vi "my ai2 and ai3 one shot on demand.vi"(0 "device name":tag="Dev1", 1 "timeout (s)":dbl=10.0 format="%0.2f", 2 "stop (T)":bool=TRUE, 11 "error in":errorcluster) -> (4 "task out":refnum<k21>, 6 "thermistor":dbl, 10 "heater":dbl, 15 "error out":errorcluster)   [LabVIEW 2019]
doc: "Creates, edits, and runs tasks using NI-DAQmx. Refer to the NI-DAQmx Readme for a complete listing of devices NI-DAQmx supports.\n\nWhen you place this Express VI on the block diagram, the DAQ Assistant launches to create a new task. After you create a task, you can double-click the DAQ Assistant Express VI to edit that task. For continuous measurement or generation, place a while loop around the DAQ Assistant Express VI."
uses:
  <vilib>/DAQmx/read.llb/DAQmx Read.vi
  <vilib>/DAQmx/read.llb/DAQmx Read (Analog 1D DBL NChan 1Samp).vi
  <vilib>/DAQmx/create/channels.llb/DAQmx Create Channel (TEDS-AI-Voltage-Basic).vi
  <vilib>/DAQmx/create/channels.llb/DAQmx Create Channel (AI-Voltage-Basic).vi
  <vilib>/DAQmx/miscellaneous.llb/DAQmx Fill In Error Info.vi
panel:
  out "data":dynamicdata(waveform)
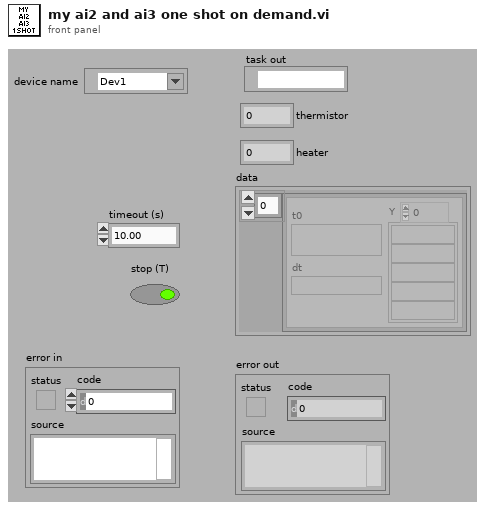
[diagram p1: front panel]
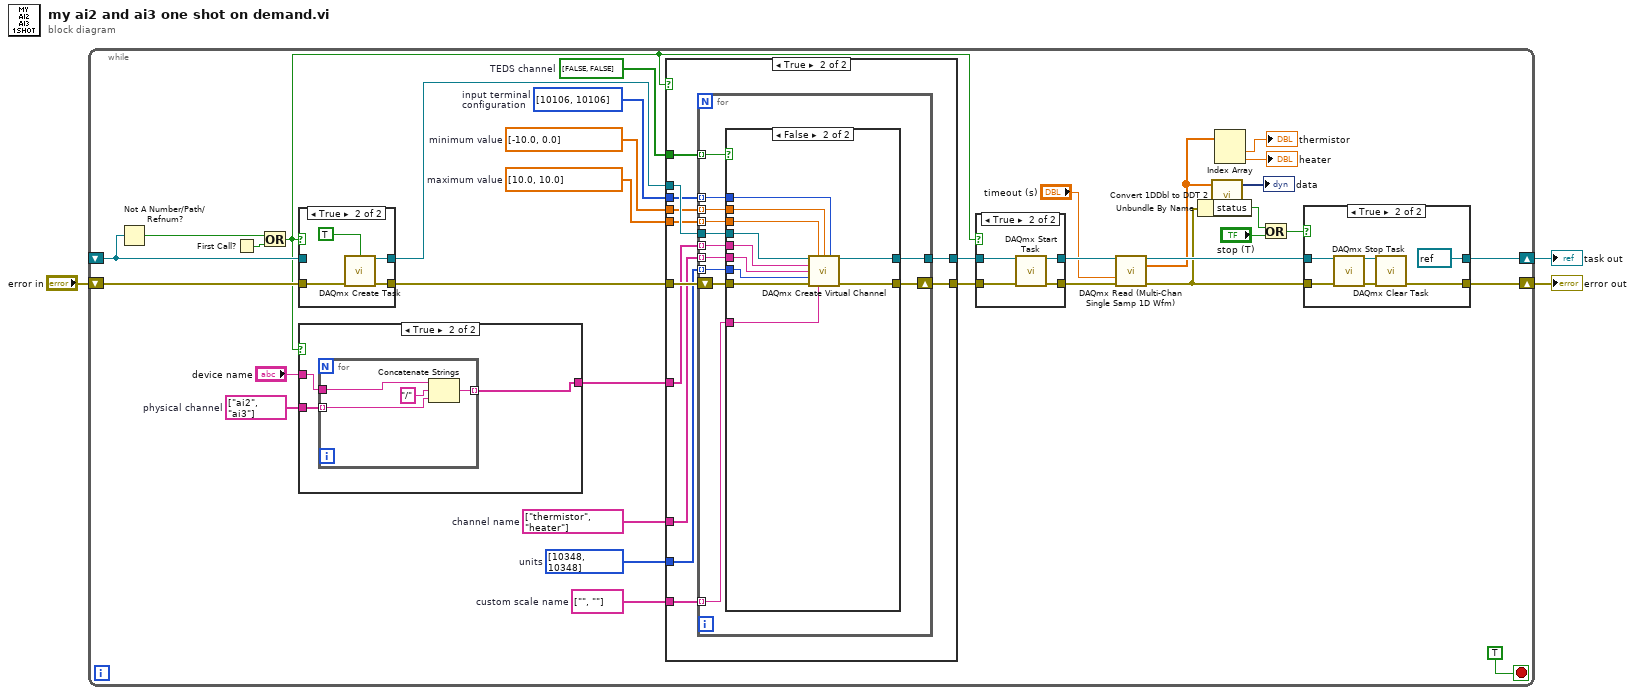
[diagram p0: block diagram]
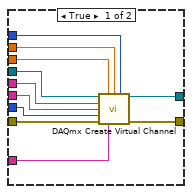
[diagram p5: hidden frame]
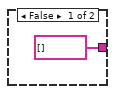
[diagram p6: hidden frame]
diagram:
  n1 = while {
    shift-right: [w13] -> w1
    shift-left: _ -> [w34]
    shift-right: [w11] -> w2
    shift-left: "error in" -> [w35]
    stop <- TRUE stop-if-true
    w21 = bool[] [FALSE, FALSE]  # TEDS channel
    w22 = string[] ["", ""]  # custom scale name
    w23 = i32[] [10348, 10348] items=["Volts"=10348, "From TEDS"=12516, "From Custom Scale"=10065]  # units
    w24 = string[] ["thermistor", "heater"]  # channel name
    w26 = dbl[] [10.0, 10.0]  # maximum value
    w27 = dbl[] [-10.0, 0.0]  # minimum value
    w28 = i32[] [10106, 10106] items=["default"=-1, "RSE"=10083, "NRSE"=10078, "Differential"=10106, "Pseudodifferential"=12529]  # input terminal configuration
    w31 = string[] ["ai2", "ai3"]  # physical channel
    n2 = Not A Number/Path/Refnum?(number/path/refnum=w34) -> (NaN/Path/Refnum?=w33:bool)
    n3 = First Call?() -> (First Call?: T/F=w36:bool)
    n4 = Or(x=w33, y=w36) -> (x .or. y?=w20:bool)
    n5 = case shown="True" w20 {
      tunnel: [w109 w113] -> w30
      tunnel: w34 -> [w109 _]
      tunnel: [w108 w112] -> w29
      tunnel: w35 -> [w108 w110]
      frame False {
      }
      frame True {
        n6 = call <vilib>:"DAQmx Create Task.vi"("auto cleanup"=TRUE, "error in"=w110) -> ("task out"=w113:refnum<k21>, "error out"=w112:errorcluster)  [unwired: 12 in]
      }
    }
    n7 = case shown="True" w20 {
      tunnel: [string[] [] w103] -> w25
      tunnel: "device name" -> [_ w102]
      tunnel: w31 -> [_ w101]
      frame False {
      }
      frame True {
        n8 = for {
          tunnel: [w107] -> w103 mode=indexing
          tunnel: w102 -> [w106]
          tunnel: w101 -> [w104] mode=indexing
          n9 = Concatenate Strings(w106, "/" ("string"), w104) -> (w107:string)
        }
      }
    }
    n10 = case shown="True" w20 {
      tunnel: [w53 w63] -> w19
      tunnel: w30 -> [w53 w65]
      tunnel: [w52 w62] -> w18
      tunnel: w29 -> [w52 w64]
      tunnel: w28 -> [_ w61]
      tunnel: w27 -> [_ w60]
      tunnel: w26 -> [_ w59]
      tunnel: w25 -> [_ w58]
      tunnel: w24 -> [_ w57]
      tunnel: w23 -> [_ w56]
      tunnel: w22 -> [_ w55]
      tunnel: w21 -> [_ w54]
      frame False {
      }
      frame True {
        n11 = for {
          tunnel: w65 -> [w77]
          tunnel: [w75] -> w63
          tunnel: w61 -> [w73] mode=indexing
          tunnel: w60 -> [w72] mode=indexing
          tunnel: w59 -> [w71] mode=indexing
          tunnel: w58 -> [w70] mode=indexing
          tunnel: w57 -> [w69] mode=indexing
          tunnel: w56 -> [w68] mode=indexing
          tunnel: w55 -> [w67] mode=indexing
          shift-right: [w74] -> w62
          shift-left: w64 -> [w76]
          tunnel: w54 -> [w66] mode=indexing
          n12 = case shown="False" w66 {
            tunnel: w77 -> [w88 w99]
            tunnel: w76 -> [w87 w98]
            tunnel: [w86 w97] -> w75
            tunnel: [w85 w96] -> w74
            tunnel: w73 -> [w84 w95]
            tunnel: w72 -> [w83 w94]
            tunnel: w71 -> [w82 w93]
            tunnel: w70 -> [w81 w92]
            tunnel: w69 -> [w80 w91]
            tunnel: w68 -> [w79 w90]
            tunnel: w67 -> [w78 w89]
            frame True {
              n13 = call-poly <vilib>:"DAQmx Create Virtual Channel.vi"("task in"=w88, "maximum value"=w82, "minimum value"=w83, "input terminal configuration"=w84, "physical channels"=w81, "name to assign"=w80, "units"=w79, "error in"=w87, "custom scale name"=w78) -> ("task out"=w86:refnum<k21>, "error out"=w85:errorcluster)  [unwired: 5 in]
            }
            frame False {
              n14 = call-poly <vilib>:"DAQmx Create Virtual Channel.vi"("task in"=w99, "maximum value"=w93, "minimum value"=w94, "input terminal configuration"=w95, "physical channels"=w92, "name to assign"=w91, "units"=w90, "error in"=w98, "custom scale name"=w89) -> ("task out"=w97:refnum<k21>, "error out"=w96:errorcluster)  [unwired: 5 in]
            }
          }
        }
      }
    }
    n15 = case shown="True" w20 {
      tunnel: [w47 w50] -> w17
      tunnel: w19 -> [w47 w51]
      tunnel: [w46 w48] -> w16
      tunnel: w18 -> [w46 w49]
      frame False {
      }
      frame True {
        n16 = call <vilib>:"DAQmx Start Task.vi"("task/channels in"=w51, "error in"=w49) -> ("task out"=w50:refnum<k21>, "error out"=w48:errorcluster)  [unwired: 12 in]
      }
    }
    n17 = call-poly "DAQmx Read (Multi-Chan Single Samp 1D Wfm).vi"("task/channels in"=w17, "timeout"="timeout (s)", "error in"=w16) -> ("task out"=w12:refnum<k21>, "data"=w6:dbl[], "error out"=w10:errorcluster)  [unwired: 10 in]
    n18 = Unbundle By Name(w10) -> ("status"=w9:bool)
    n19 = call <vilib>:"Convert 1DDbl to DDT 2.vi"("Array"=w6) -> ("Dynamic Data Type"=→"data":dynamicdata)  [unwired: 3 in]
    n20 = Index Array(array=w6) -> (element #1=→"thermistor":dbl, element #2=→"heater":dbl)  [unwired: 2 in]
    n21 = Or(x=w9, y="stop (T)") -> (x .or. y?=w7:bool)
    n22 = case shown="True" w7 {
      tunnel: [w39 refnum<k21> refnum ("task in")] -> w13
      tunnel: w12 -> [w39 w45]
      tunnel: [w38 w42] -> w11
      tunnel: w10 -> [w38 w44]
      frame False {
      }
      frame True {
        n23 = call <vilib>:"DAQmx Stop Task.vi"("task/channels in"=w45, "error in"=w44) -> ("task out"=w41:refnum<k21>, "error out"=w43:errorcluster)  [unwired: 12 in]
        n24 = call <vilib>:"DAQmx Clear Task.vi"("task in"=w41, "error in"=w43) -> ("error out"=w42:errorcluster)  [unwired: 13 in]
      }
    }
  }
  "error out" <- w2
  "task out" <- w1
